vi "smart controller.vi"() -> ()   [LabVIEW 2014]
uses:
  <vilib>/Instr/_visa.llb/VISA Configure Serial Port (Instr).vi
  Environmental Chamber LabVIEW and Instruments/Drivers and Software/Keithley 2100 Series/Public/Configure/Configure 2 Wire Resistance.vi
  <vilib>/Utility/file.llb/Write To Spreadsheet File (string).vi
  Environmental Chamber LabVIEW and Instruments/Drivers and Software/keithley_6430/Keithley 6430/Public/Data/Read (Single Point).vi
  Environmental Chamber LabVIEW and Instruments/Drivers and Software/LabVIEW 8.2 Drivers/keithley_24xx/Keithley 24XX/Public/Data/Read (Single Point).vi
  <vilib>/Utility/file.llb/Read From Spreadsheet File (string).vi
  Environmental Chamber LabVIEW and Instruments/Drivers and Software/keithley_24xx/Keithley 24XX/Keithley 24XX.lvlib
  Environmental Chamber LabVIEW and Instruments/Drivers and Software/keithley_6430/Keithley 6430/Keithley 6430.lvlib
  Environmental Chamber LabVIEW and Instruments/Drivers and Software/Keithley 2100 Series/Keithley 2100 Series.lvlib
panel:
  in  "Smart start":T1={"set signal change"=100.0, " Begin smart start"=FALSE, "Reference signal"=enum."Keithley 2420", " smart start running"=FALSE} {"set signal change" min=0.0 max=100.0 step=5.0 format="%#_2f"}
  out "saving data?":bool
  out "ArduinoQCM\ncluster":T2 caption="OpenQCM" {"Freq 5" format="%#_10g"; "Freq 4" format="%#_10g"; "Freq 3" format="%#_10g"; "Freq 2" format="%#_10g"; "Freq 1" format="%#_10g"}
  in  "Data logging settings":T3={"Save during sequence only"=TRUE, "Save now"=FALSE, "sec between data points"=0.0, "Current data file path"=path "", "Save sample names"={"QCM1"="aQCM2", "QCM2"="aQCM2", "QCM3"="aQCM3", "QCM4"="aQCM4", "QCM5"="aQCM5", "QCM6"="aQCM6", "SRS"="sample_SRS", "K-2420"="Keithley2420", "K-6430"="Keithley6430", "K-2100"="Keithley2100"}, "Experiment Notes"=""} {"sec between data points" min=0.0 max=30.0 format="%#_13g"}
  in  "Sequence cluster":T4={"Save sequence"=FALSE, "Clear sequence"=FALSE, "Import sequence file"=FALSE, "Tare elapsed time"=TRUE, "Run Sequence"=FALSE, "Stop program when sequence ends"=TRUE, "User-defined\nsequence"=[], "Sequence end time"="", "Sequence\npreview"=[], "Current\nstep"=0, "Jump to next step"=FALSE} caption="Sequence settings"
  in  "Pressure parameters cluster":T5={"valve % open"=100.0, "Desired pressure"=0.0, "Vapor sccm"=0.0, "Gas sccm"=0.0, "Valve mode"=enum."% Open", "Pressure Mode"=enum."Abs. pressure", "analyte partial pressure"=23.8, "Turbo pump\nauto on"=TRUE, "Valve position (%)"=0.0, "read pressure"=0.0, "read vapor flow"=0.0, "read gas flow"=0.0, "pressure chart"={"pressure"=0.0}} caption="Pressure settings" {"read gas flow" format="%#_3g"; "read vapor flow" format="%#_3g"; "read pressure" format="%#_7f"; "Valve position (%)" format="%#_3g"; "analyte partial pressure" min=0.0 max=100.0 step=5.0; "Gas sccm" min=0 max=200 step=5; "Vapor sccm" min=0 max=200 step=5; "Desired pressure" min=0.0 max=760.0 step=5.0; "valve % open" min=0.0 max=100.0 step=5.0 format="%#_2f"}
  out "J-KEM temp chart":dbl(graph)
  out "Elapsed time (min)":dbl
  out "State date/time":string caption="Start time"
  out "K-2100 (Ohm)":cluster{"Measurement":dbl}(graph) caption="K-2100 Ohm"
  out "K-6430":cluster{"Measurement":dbl}(graph)
  out "K-2420":cluster{"Resistance":sgl}(graph)
  in  "Gate time (sec)":enum16{"0.1", "1.0 ", "10"}(ring)=enum."1.0 "
  out "MHz":dbl format="%.9f"
  out "QCM plot":T6(graph)
  in  "Stop":bool
  in  "Clear all charts":bool
  out "O2 sensor output":dbl[](array[numeric]) caption="atm\nTorr"
  in  "rapidox O2 Sensor":bool
  in  "setnag O2 Pump":bool
  in  "Baud Rate 2":i32(ring)=2 items=["2400", "4800", "9600", "19200", "38400", "57600", "115200"]
  in  "Com Port":i32(ring) items=["Com 1", "Com 2", "Com 3", "Com 4", "Com 5", "Com 6", "COM 7", "COM 8", "COM 9", "COM 10", "COM 11", "COM 12", "com 13", "COM 14"]
  in  "Com Port 2":i32(ring) items=["Com 1", "Com 2", "Com 3", "Com 4", "Com 5", "Com 6", "COM 7", "COM 8", "COM 9", "COM 10", "COM 11", "COM 12", "com 13", "COM 14"]
  out "Waveform Chart":cluster{dbl}(graph)
  out "O2 Concentration (PPM)":dbl
  out "Waveform Chart 6":cluster{dbl}(graph)
  # "Currently Unused"
  # "signal changes by less than"
  # "units"
  # "Run sequence when"
  # "100%"
  # "SRS"
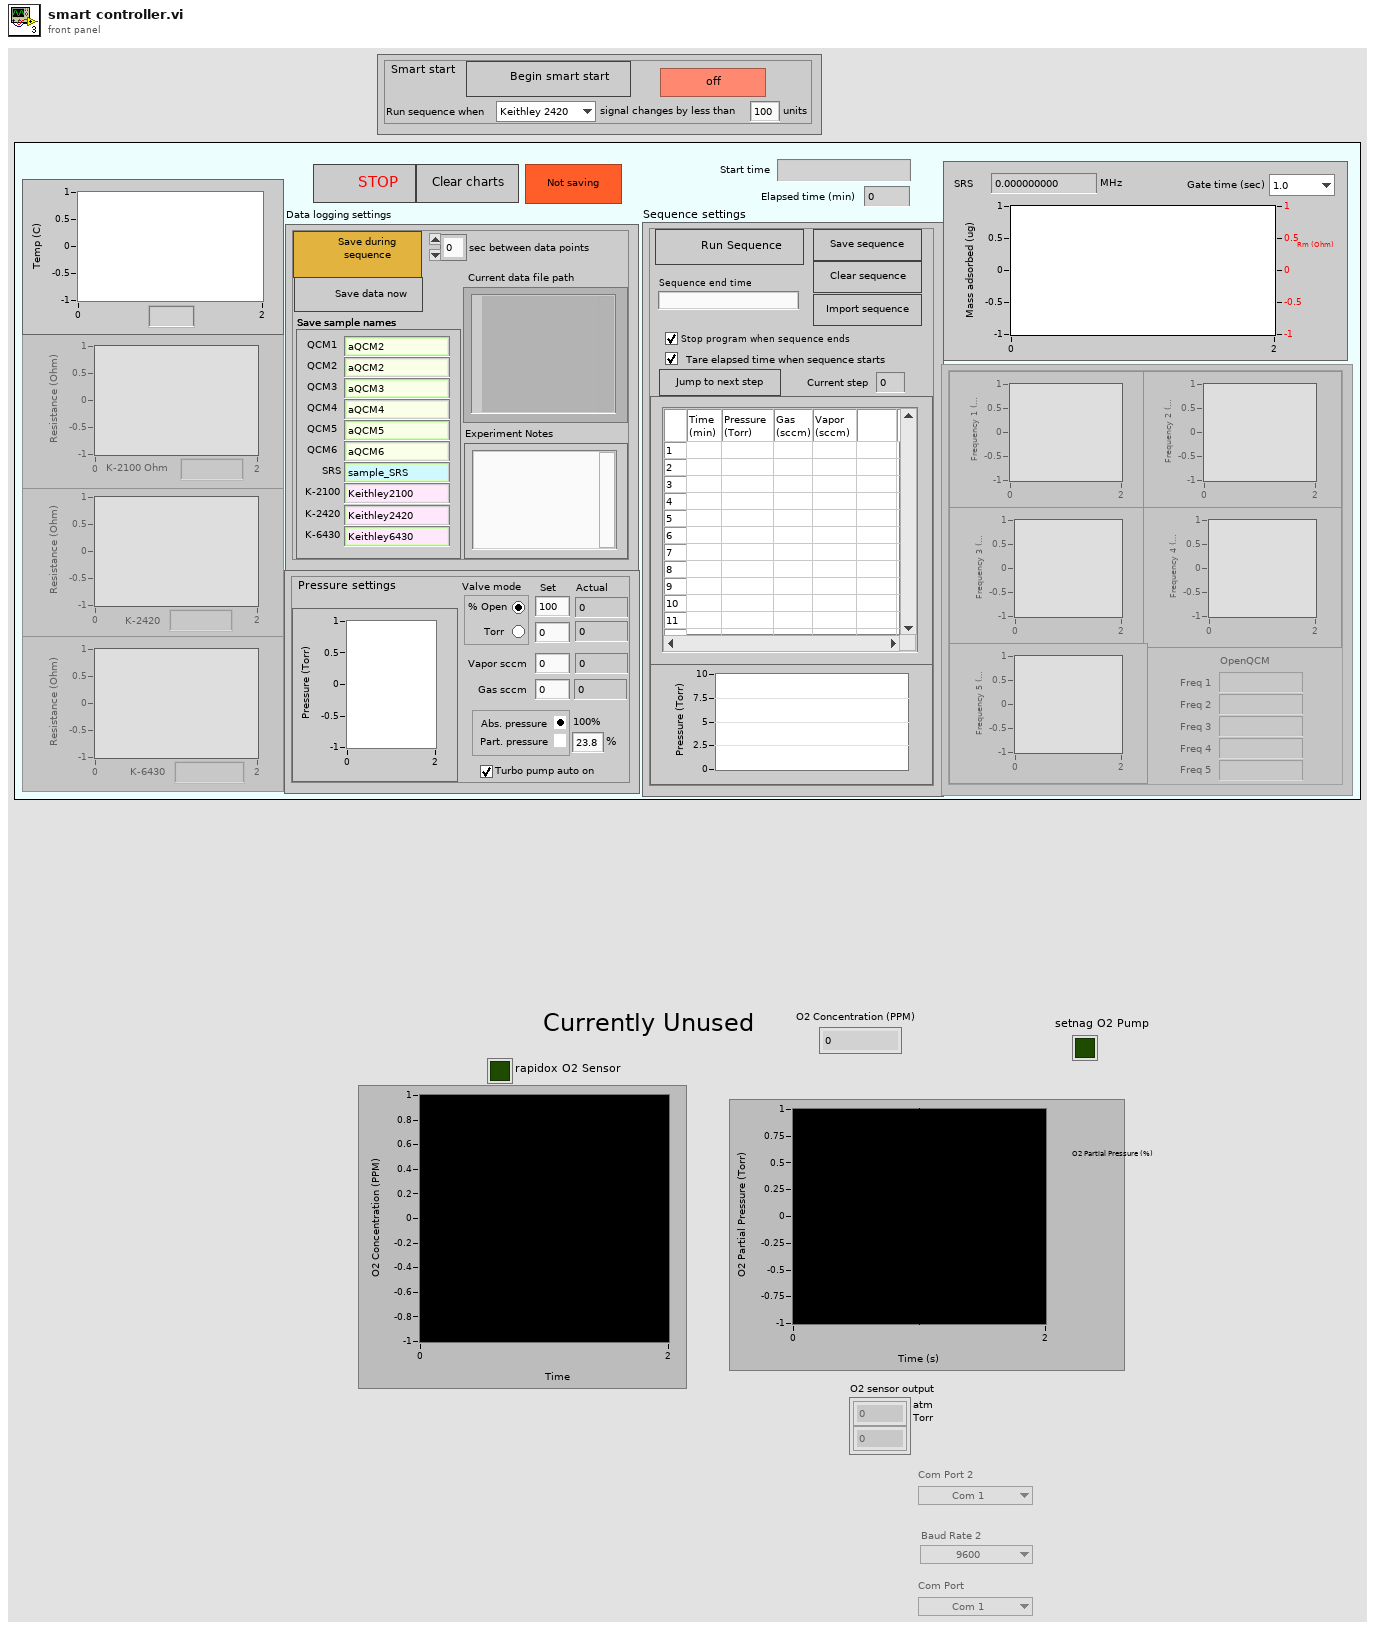
[diagram p1: front panel]
types:
  T1 = cluster{"set signal change":dbl, " Begin smart start":bool, "Reference signal":enum16{"SRS QCM", "Keithley 2420", "Keithley 6430"}, " smart start running":bool}
  T2 = cluster{"arduino qcm 1":dbl, "Freq 1":dbl, "arduino qcm 2":dbl, "Freq 2":dbl, "arduino qcm 3":dbl, "Freq 3":dbl, "arduino qcm 4":dbl, "Freq 4":dbl, "arduino qcm 5":dbl, "Freq 5":dbl}
  T3 = cluster{"Save during sequence only":bool, "Save now":bool, "sec between data points":dbl, "Current data file path":path, "Save sample names":cluster{"QCM1":string, "QCM2":string, "QCM3":string, "QCM4":string, "QCM5":string, "QCM6":string, "SRS":string, "K-2420":string, "K-6430":string, "K-2100":string}, "Experiment Notes":string}
  T4 = cluster{"Save sequence":bool, "Clear sequence":bool, "Import sequence file":bool, "Tare elapsed time":bool, "Run Sequence":bool, "Stop program when sequence ends":bool, "User-defined\nsequence":string[][], "Sequence end time":string, "Sequence\npreview":cluster{dbl[], dbl[]}[], "Current\nstep":i32, "Jump to next step":bool}
  T5 = cluster{"valve % open":dbl, "Desired pressure":dbl, "Vapor sccm":sgl, "Gas sccm":sgl, "Valve mode":enum32{"% Open", "Torr "}, "Pressure Mode":enum32{"Abs. pressure", " Part. pressure"}, "analyte partial pressure":dbl, "Turbo pump\nauto on":bool, "Valve position (%)":dbl, "read pressure":dbl, "read vapor flow":dbl, "read gas flow":dbl, "pressure chart":cluster{"pressure":dbl}}
  T6 = cluster{"Numeric Control":dbl, "Resistance out":dbl}
  T7 = cluster{"Keithley 6430":bool, "J-KEM":bool, "Keithley 2420":bool, "Keithley 2100":bool, "SRS QCM":bool, "Pressure control":bool, "Arduino":bool}
  T8 = enum8{"Enabled", "Disabled", "Disabled and Grayed Out"}
  T9 = cluster{"Arduino 1":refnum<visa-resource-name>, "Arduino 2":refnum<visa-resource-name>, "Arduino 3":refnum<visa-resource-name>, "Arduino 4":refnum<visa-resource-name>, "Arduino 5":refnum<visa-resource-name>}
  T10 = enum16{"open", "open or create", "create or replace", "create", "open (read only)"}
  T11 = enum16{"no parity", "odd parity", "even parity", "mark parity", "space parity"}
  T12 = cluster{"f":dbl, "f":dbl, "f":dbl, "f":dbl, "f":dbl}
  T13 = cluster{"String":string, "String":string, "String":string}
  T14 = cluster{"task out":refnum<k21>, "error out":errorcluster, "task out":refnum<k21>, "error out":errorcluster, "task out":refnum<k21>, "error out":errorcluster, "VISA resource name":refnum<visa-resource-name>, "error out":errorcluster}
  T15 = cluster{"task out":refnum<k21>, "error out":errorcluster, "task out":refnum<k21>, "error out":errorcluster, "task out":refnum<k21>, "error out":errorcluster, "VISA resource name out":refnum<visa-resource-name>, "error out":errorcluster}
  T16 = cluster{bool, "VISA resource name":refnum<visa-resource-name>, "error out":errorcluster}
  T17 = cluster{bool, "VISA resource name out":refnum<visa-resource-name>, "error out":errorcluster}
  T18 = cluster{"VISA resource name out":refnum<visa-resource-name>, "error out":errorcluster, "VISA resource name out":refnum<visa-resource-name>, "error out":errorcluster, "VISA resource name out":refnum<visa-resource-name>, "error out":errorcluster, "VISA resource name out":refnum<visa-resource-name>, "error out":errorcluster, "VISA resource name out":refnum<visa-resource-name>, "error out":errorcluster}
  T19 = cluster{bool, cluster{"task out":refnum<k21>, "error out":errorcluster, "task out":refnum<k21>, "error out":errorcluster, "task out":refnum<k21>, "error out":errorcluster, "VISA resource name out":refnum<visa-resource-name>, "error out":errorcluster}}
  T20 = cluster{"Boolean":bool, "VISA resource name out":refnum<visa-resource-name>, "error out":errorcluster}
  T21 = cluster{bool, "VISA out":refnum<visa-resource-name>, "error out":errorcluster}
  T22 = cluster{"Boolean":bool, "VISA out":refnum<visa-resource-name>, "error out":errorcluster}
  T23 = cluster{"Numeric Control":dbl, "Cluster":cluster{"Numeric Control":dbl}, "String":string, "error out":errorcluster}
  T24 = cluster{bool, "Com Port":i32, "Numeric Control out":dbl}
  T25 = cluster{"VISA Refnum out":refnum<visa-resource-name>, "error out":errorcluster, "VISA Refnum out":refnum<visa-resource-name>, "error out":errorcluster, "VISA Refnum out":refnum<visa-resource-name>, "error out":errorcluster, "VISA Refnum out":refnum<visa-resource-name>, "error out":errorcluster, "VISA Refnum out":refnum<visa-resource-name>, "error out":errorcluster}
  T26 = cluster{"f":string, "f":string, "f":string, "f":string, "f":string}
  T27 = cluster{"String data out":string, string, string, string}
  T28 = cluster{"valve % open":dbl, "Desired pressure":dbl, "Vapor sccm":sgl, "Gas sccm":sgl, "Valve mode":enum32{"% Open", "Torr "}, "Pressure Mode":enum32{"Abs. pressure", " Part. pressure"}, "analyte partial pressure":dbl, "Turbo pump\nauto on":bool}
  T29 = cluster{"User-defined\nsequence":string[][], "Present (s)":dbl, "current  step # in":i32, "sequence end time in":timestamp}
  T30 = cluster{"current  step # in":i32, "sequence end time in":timestamp, "Boolean":bool}
  T31 = cluster{"press/RH/gas/vapor":cluster{"pressure":string, "RH":string, "gas flow":string, "vapor flow":string}, "Cluster":cluster{"Valve position (%)":dbl, "read pressure":dbl, "read vapor flow":dbl, "read gas flow":dbl}}
  T32 = cluster{"Boolean":bool, "DAQ IDs in":cluster{"task out":refnum<k21>, "error out":errorcluster, "task out":refnum<k21>, "error out":errorcluster, "task out":refnum<k21>, "error out":errorcluster, "VISA Refnum out":refnum<visa-resource-name>, "error out":errorcluster}}
  T33 = cluster{"f":dbl, "f":dbl, "f":dbl, "f":dbl, "f":dbl}[]
  T34 = cluster{"pressure":string, "RH":string, "gas flow":string, "vapor flow":string}
  T35 = cluster{"Valve position (%)":dbl, "read pressure":dbl, "read vapor flow":dbl, "read gas flow":dbl}
  T36 = cluster{"f":dbl, "f":dbl, "f":dbl, "f":dbl, "f":dbl, "f":dbl, "f":dbl, "f":dbl, "f":dbl, "f":dbl}
  T37 = cluster{"QCM1":string, "QCM2":string, "QCM3":string, "QCM4":string, "QCM5":string, "QCM6":string, "SRS":string, "K-2420":string, "K-6430":string, "K-2100":string}
  T38 = cluster{"task out":refnum<k21>, "error out":errorcluster, "task out":refnum<k21>, "error out":errorcluster, "task out":refnum<k21>, "error out":errorcluster, "VISA Refnum out":refnum<visa-resource-name>, "error out":errorcluster}
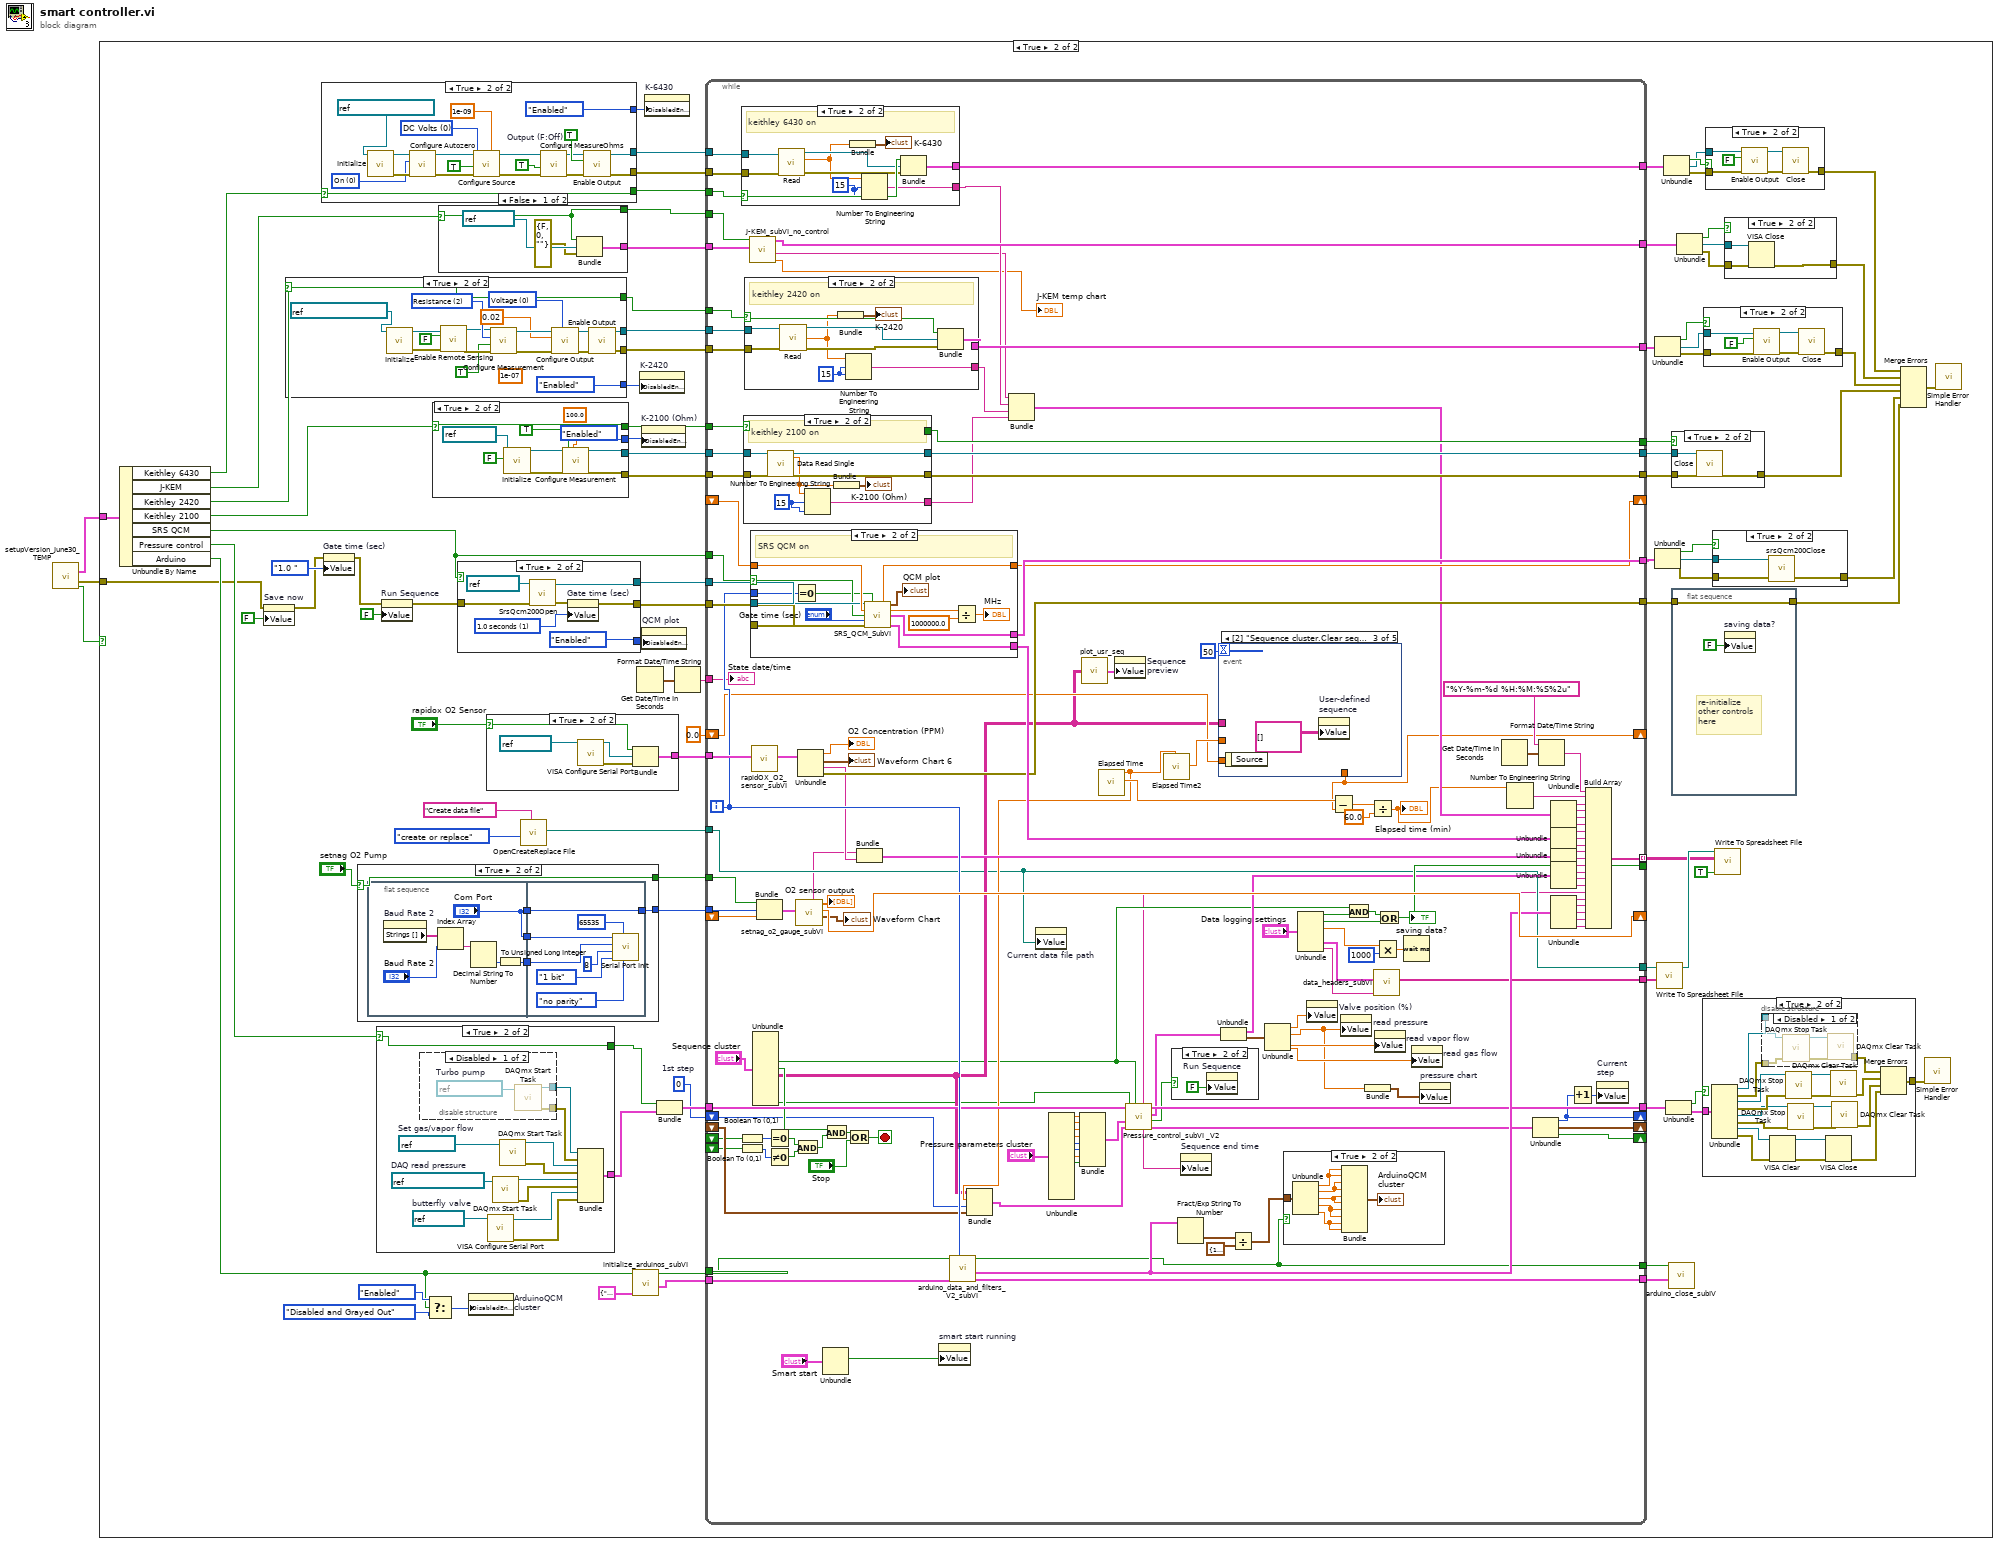
[diagram p0: block diagram]
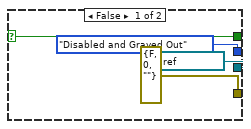
[diagram p4: hidden frame]
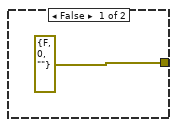
[diagram p5: hidden frame]
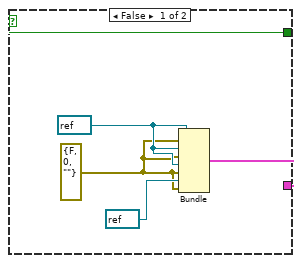
[diagram p7: hidden frame]
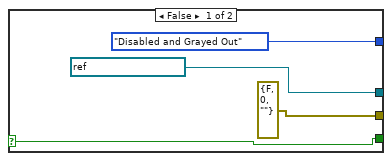
[diagram p10: hidden frame]
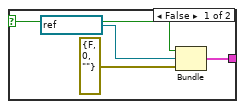
[diagram p11: hidden frame]
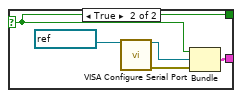
[diagram p13: hidden frame]
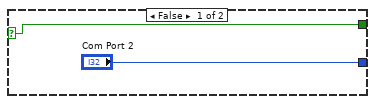
[diagram p14: hidden frame]
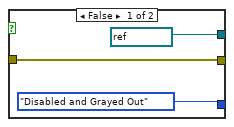
[diagram p16: hidden frame]
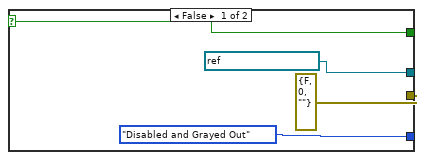
[diagram p18: hidden frame]
diagram:
  n1 = call "setupVersion_June30_TEMP.vi"() -> ("Instruments on/off"=w1:T7, "error IO"=w2:errorcluster, "OK"=w3:bool)  [unwired: 13 in]
  n2 = case shown="True" w3 {
    tunnel: w2 -> [_ w8]
    tunnel: w1 -> [_ w16]
    frame False {
    }
    frame True {
      w28 = 0  # 1st step
      n3 = Unbundle By Name(w16) -> ("Keithley 6430"=w15:bool, "J-KEM"=w14:bool, "Keithley 2420"=w13:bool, "Keithley 2100"=w12:bool, "SRS QCM"=w11:bool, "Pressure control"=w10:bool, "Arduino"=w9:bool)
      n4 = property on="Save now" class="Bool (strict)"(error in=w8, "Value"=FALSE) -> (error out=w7:errorcluster)  [unwired: 1 in, 1 out]
      n5 = case shown="True" w13 {
        selector: w13 -> [w255 w259]
        tunnel: [refnum<visa-resource-name> "GPIB1::24::INSTR" ("VISA resource name") w268] -> w92
        tunnel: [errorcluster {"status"=FALSE, "code"=0, "source"=""} ("error out") w263] -> w91
        tunnel: [T8."Disabled and Grayed Out" ("Disabled") T8."Enabled" ("Disabled")] -> w55
        tunnel: [w255 w259] -> w48
        frame False {
        }
        frame True {
          (unwired) 1e-07 ("Manual Range (1.0)")
          w270 = u16 0 items=["Voltage", "Current"] ("Source Mode  (0: Voltage)")
          w275 = u16 2 items=["Volts", "Current", "Resistance"] ("Function (0: Volts)")
          n6 = call "Initialize.vi"("VISA resource name"=refnum<visa-resource-name> "GPIB1::24::INSTR") -> ("error out"=w264:errorcluster, "VISA resource name out"=w267:refnum<visa-resource-name>)  [unwired: 9 in]
          n7 = call "Enable Remote Sensing.vi"("error in (no error)"=w264, "Enable Remote Sensing (T: Enable)"=FALSE ("4-wire?"), "VISA resource name"=w267) -> ("error out"=w265:errorcluster, "VISA resource name out"=w266:refnum<visa-resource-name>)  [unwired: 7 in]
          n8 = call "Configure Measurement.vi"("error in (no error)"=w265, "Enable Auto Range (T:Enable)"=TRUE, "Function (0: Volts)"=w275, "VISA resource name"=w266) -> ("error out"=w274:errorcluster, "VISA resource name out"=w273:refnum<visa-resource-name>)  [unwired: 6 in]
          n9 = call "Configure Output.vi"("Source Mode  (0: Voltage)"=w270, "error in (no error)"=w274, "Output Level (0)"=0.02 ("Applied Voltage (V)"), "VISA resource name"=w273) -> ("error out"=w272:errorcluster, "VISA resource name out"=w271:refnum<visa-resource-name>)  [unwired: 6 in]
          n10 = call "Enable Output.vi"("error in (no error)"=w272, "VISA resource name"=w271) -> ("error out"=w263:errorcluster, "VISA resource name out"=w268:refnum<visa-resource-name>)  [unwired: 8 in]
        }
      }
      n11 = case shown="True" w15 {
        selector: w15 -> [w169 w173]
        tunnel: [refnum<visa-resource-name> "GPIB0::29::INSTR" ("VISA resource name") w186] -> w61
        tunnel: [errorcluster {"status"=FALSE, "code"=0, "source"=""} ("error out") w187] -> w60
        tunnel: [T8."Disabled and Grayed Out" ("Disabled") T8."Enabled" ("Disabled")] -> w54
        tunnel: [w169 w173] -> w47
        frame False {
        }
        frame True {
          w175 = u16 0 items=["DC Volts", "DC Current"] ("Source Function (0: DC Volts)")
          w182 = u16 0 items=["On", "Off", "Once"] ("Autozero  (0: On)")
          w190 = TRUE  # Output (F:Off)
          n12 = call "Initialize.vi"("VISA resource name"=refnum<visa-resource-name> "GPIB0::30::INSTR") -> ("error out"=w183:errorcluster, "VISA resource name out"=w184:refnum<visa-resource-name>)  [unwired: 4 in, 5 out]
          n13 = call "Configure Autozero.vi"("error in (no error)"=w183, "Autozero  (0: On)"=w182, "VISA resource name"=w184) -> ("error out"=w178:errorcluster, "VISA resource name out"=w180:refnum<visa-resource-name>)  [unwired: 7 in]
          n14 = call "Configure Source.vi"("I-Source Level [A]"=1e-09, "error in (no error)"=w178, "Auto Range (T:Enable)"=TRUE, "Source Function (0: DC Volts)"=w175, "VISA resource name"=w180) -> ("error out"=w177:errorcluster, "VISA resource name out"=w179:refnum<visa-resource-name>)  [unwired: 5 in]
          n15 = call "Configure MeasureOhms.vi"("error in (no error)"=w177, "Auto Range (T:Enable)"=TRUE, "VISA resource name"=w179) -> ("error out"=w191:errorcluster, "VISA resource name out"=w189:refnum<visa-resource-name>)  [unwired: 3 in, 4 out]
          n16 = call "Enable Output.vi"("error in (no error)"=w191, "Enable Output (F:Off)"=w190, "VISA resource name"=w189) -> ("error out"=w187:errorcluster, "VISA resource name out"=w186:refnum<visa-resource-name>)  [unwired: 7 out]
        }
      }
      n17 = property on="Gate time (sec)" class="Enum (strict)"(error in=w7, "Value"=enum16{"0.1", "1.0 ", "10"}."1.0 " ("Gate time (sec)")) -> (error out=w17:errorcluster)  [unwired: 1 in, 1 out]
      n18 = case shown="True" "setnag O2 Pump" {
        selector: "setnag O2 Pump" -> [w214 w216]
        tunnel: ["Com Port 2" w217] -> w88
        tunnel: [w214 w216] -> w36
        frame False {
        }
        frame True {
          n19 = flat-sequence {
            tunnel: ["Com Port"] -> w220
            tunnel: [w222] -> w219
            tunnel: ["Com Port"] -> w218
            tunnel: w220 -> [w228]
            tunnel: w219 -> [w227]
            tunnel: w218 -> [w229]
            tunnel: [w229] -> w217
            frame #0 {
              n20 = property on="Baud Rate 2" class="Ring (strict)"() -> ("Strings []"=w224:string[])  [unwired: 2 in, 2 out]
              n21 = Index Array(array=w224, index="Baud Rate 2") -> (element=w225:string)
              n22 = Decimal String To Number(string=w225) -> (number=w223:i32)  [unwired: 2 in, 1 out]
              n23 = To Unsigned Long Integer(number=w223) -> (unsigned 32bit integer=w222:u32)
            }
            frame #1 {
              n24 = call <vilib>:"Serial Port Init.vi"("parity"=T11."no parity", "buffer size"=u16 65535, "stop bits"=enum16{"1 bit", "1.5 bits", "2 bits"}."1 bit", "data bits"=u16 8, "baud rate"=w227, "port number"=w228) -> ()  [unwired: 1 in, 1 out]
            }
          }
        }
      }
      n25 = case shown="True" w10 {
        selector: w10 -> [w141 w146]
        tunnel: [w142 w148] -> w30
        tunnel: [w141 w146] -> w31
        frame False {
          w144 = refnum<k21> refnum ("task out")
          w143 = errorcluster {"status"=FALSE, "code"=0, "source"=""} ("error out")
          n26 = Bundle("task out"=w144, "error out"=w143, "task out"=w144, "error out"=w143, "task out"=w144, "error out"=w143, "VISA resource name"=refnum<visa-resource-name> refnum, "error out"=w143) -> (w142:T14)  [unwired: 1 in]
        }
        frame True {
          w156 = refnum<visa-resource-name> "COM5"  # butterfly valve
          w157 = refnum<k21> "Setflow"  # Set gas/vapor flow
          w158 = refnum<k21> "AllDaqReadings"  # DAQ read pressure
          n27 = disable-structure shown="Disabled" {
            disable-tunnel: [w160 _] -> w155
            disable-tunnel: [w159 _] -> w154
            frame Disabled {
              w161 = refnum<k21> "TurboON"  # Turbo pump
              n28 = call <vilib>:"DAQmx Start Task.vi"("task/channels in"=w161) -> ("task out"=w160:refnum<k21>, "error out"=w159:errorcluster)  [unwired: 13 in]
            }
            frame Enabled {
            }
          }
          n29 = call-poly "VISA Configure Serial Port"("VISA resource name"=w156) -> ("VISA resource name out"=w149:refnum<visa-resource-name>, "error out"=w147:errorcluster)  [unwired: 13 in]
          n30 = call <vilib>:"DAQmx Start Task.vi"("task/channels in"=w158) -> ("task out"=w151:refnum<k21>, "error out"=w150:errorcluster)  [unwired: 13 in]
          n31 = call <vilib>:"DAQmx Start Task.vi"("task/channels in"=w157) -> ("task out"=w153:refnum<k21>, "error out"=w152:errorcluster)  [unwired: 13 in]
          n32 = Bundle("task out"=w155, "error out"=w154, "task out"=w153, "error out"=w152, "task out"=w151, "error out"=w150, "VISA resource name out"=w149, "error out"=w147) -> (w148:T15)  [unwired: 1 in]
        }
      }
      n33 = property on="Run Sequence" class="Bool (strict)"(error in=w17, "Value"=FALSE) -> (error out=w23:errorcluster)  [unwired: 1 in, 1 out]
      n34 = Select(t=T8."Enabled" ("Disabled"), s=w9, f=T8."Disabled and Grayed Out" ("Disabled")) -> (s? t:f=w22:T8)
      n35 = case shown="True" w12 {
        selector: w12 -> [w102 w108]
        tunnel: [refnum<visa-resource-name> "K-2100" ("VISA resource name out") w111] -> w45
        tunnel: [errorcluster {"status"=FALSE, "code"=0, "source"=""} ("error out") w110] -> w44
        tunnel: [w102 w108] -> w43
        tunnel: [T8."Disabled and Grayed Out" ("Disabled") T8."Enabled" ("Disabled")] -> w38
        frame False {
        }
        frame True {
          n36 = call "Initialize.vi"("VISA resource name"=refnum<visa-resource-name> "K-2100", "Reset? (T: Reset)"=FALSE) -> ("VISA resource name out"=w112:refnum<visa-resource-name>, "error out"=w109:errorcluster)  [unwired: 16 in]
          n37 = call-poly "Configure Measurement.vi"("VISA resource name"=w112, "error in (no error)"=w109, "Auto Range? (T: Auto)"=TRUE, "Custom Range (100 Ohm)"=100.0 ("Temp (C) 2")) -> ("VISA resource name out"=w111:refnum<visa-resource-name>, "error out"=w110:errorcluster)  [unwired: 14 in]
        }
      }
      n38 = case shown="False" w14 {
        selector: w14 -> [w205 w210]
        tunnel: [w206 w211] -> w77
        tunnel: [w205 w210] -> w71
        frame False {
          n39 = Bundle(w205, "VISA resource name"=refnum<visa-resource-name> "COM3", "error out"=errorcluster {"status"=FALSE, "code"=0, "source"=""}) -> (w206:T16)  [unwired: 1 in]
        }
        frame True {
          n40 = call-poly "VISA Configure Serial Port"("VISA resource name"=refnum<visa-resource-name> "COM3") -> ("VISA resource name out"=w212:refnum<visa-resource-name>, "error out"=w209:errorcluster)  [unwired: 13 in]
          n41 = Bundle(w210, "VISA resource name out"=w212, "error out"=w209) -> (w211:T17)  [unwired: 1 in]
        }
      }
      n42 = case shown="True" w11 {
        tunnel: [refnum<visa-resource-name> "COM6" ("VISA in") w244] -> w90
        tunnel: [w239 w241] -> w89
        tunnel: w23 -> [w239 w246]
        tunnel: [T8."Disabled and Grayed Out" ("Disabled") T8."Enabled" ("Disabled")] -> w56
        frame False {
        }
        frame True {
          w243 = u16 1 items=["0.1 seconds", "1.0 seconds", "10.0 seconds"] ("Gate time")
          n43 = call "SrsQcm200Open.vi"("error in"=w246, "VISA in"=refnum<visa-resource-name> "COM6") -> ("error out"=w242:errorcluster, "VISA out"=w244:refnum<visa-resource-name>)  [unwired: 3 in]
          n44 = property on="Gate time (sec)" class="Enum (strict)"(error in=w242, "Value"=w243) -> (error out=w241:errorcluster)  [unwired: 1 in, 1 out]
        }
      }
      n45 = property on="ArduinoQCM\ncluster" class="Clust (strict)"("DisabledEnum"=w22) -> ()  [unwired: 2 in, 2 out]
      n46 = case shown="True" "rapidox O2 Sensor" {
        selector: "rapidox O2 Sensor" -> [w192 w197]
        tunnel: [w193 w198] -> w67
        frame False {
          n47 = Bundle(w192, "VISA resource name"=refnum<visa-resource-name> "COM7", "error out"=errorcluster {"status"=FALSE, "code"=0, "source"=""}) -> (w193:T16)  [unwired: 1 in]
        }
        frame True {
          n48 = call-poly "VISA Configure Serial Port"("VISA resource name"=refnum<visa-resource-name> "COM7") -> ("VISA resource name out"=w199:refnum<visa-resource-name>, "error out"=w196:errorcluster)  [unwired: 13 in]
          n49 = Bundle(w197, "VISA resource name out"=w199, "error out"=w196) -> (w198:T17)  [unwired: 1 in]
        }
      }
      n50 = call "OpenCreateReplace File.vi"("prompt"="Create data file", "function (open:0)"=T10."create or replace") -> ("new file path"=w46:path)  [unwired: 6 in, 3 out]
      n51 = call "initialize_arduinos_subVI.vi"("arduino 1-6 addresses"=T9 {"Arduino 1"="COM21", "Arduino 2"="COM22", "Arduino 3"="COM23", "Arduino 4"="COM24", "Arduino 5"="COM26"}, "arduinos on?"=w9) -> ("arduino addresses/errors"=w32:T18, "arduinos on/off"=w52:bool)  [unwired: 8 in]
      n52 = Get Date/Time In Seconds() -> (seconds since 1Jan1904=w94:timestamp)
      n53 = property on="K-2420" class="WFChart (strict)"("DisabledEnum"=w55) -> ()  [unwired: 2 in, 2 out]
      n54 = property on="K-2100 (Ohm)" class="WFChart (strict)"("DisabledEnum"=w38) -> ()  [unwired: 2 in, 2 out]
      n55 = property on="QCM plot" class="WFChart (strict)"("DisabledEnum"=w56) -> ()  [unwired: 2 in, 2 out]
      n56 = property on="K-6430" class="WFChart (strict)"("DisabledEnum"=w54) -> ()  [unwired: 2 in, 2 out]
      n57 = Bundle(w31, w30) -> (w29:T19)  [unwired: 1 in]
      n58 = Format Date/Time String(seconds (now)=w94) -> (date/time string=w35:string)  [unwired: 2 in]
      n59 = while {
        shift-right: [w423] -> _
        shift-left: _ -> [w345]
        tunnel: [w407] -> w53 mode=indexing if=w371
        tunnel: w48 -> [w412]
        tunnel: w92 -> [w422]
        tunnel: w91 -> [w421]
        tunnel: w90 -> [w420]
        tunnel: w89 -> [w419]
        tunnel: w11 -> [w418]
        tunnel: w36 -> [w347]
        tunnel: w88 -> [w348]
        tunnel: [w417] -> w85
        tunnel: [w416] -> w81
        tunnel: w77 -> [w415]
        tunnel: [w414] -> w76
        tunnel: w71 -> [w413]
        tunnel: w67 -> [w359]
        tunnel: [w355] -> w5
        tunnel: [w287] -> w66
        tunnel: w46 -> [w287]
        shift-right: [w405] -> _
        shift-left: _ -> [w406]
        tunnel: w61 -> [w411]
        tunnel: w60 -> [w410]
        tunnel: [w409] -> w59
        tunnel: [w371] -> _
        tunnel: w52 -> [w354]
        tunnel: w32 -> [w398]
        tunnel: [w353] -> w50
        tunnel: [w397] -> w51
        tunnel: [w390] -> w49
        tunnel: w47 -> [w383]
        tunnel: w45 -> [w370]
        tunnel: w44 -> [w369]
        tunnel: w43 -> [w368]
        tunnel: [w367] -> w42
        tunnel: [w366] -> w41
        tunnel: [w365] -> w40
        shift-right: [w339] -> _
        shift-left: 0.0 ("Elapsed Time (s)") -> [w340]
        tunnel: w35 -> [w330]
        tunnel: w29 -> [w312]
        shift-right: [w282] -> _
        shift-left: w28 -> [w301]
        shift-right: [w307] -> _
        shift-left: _ -> [w305]
        shift-right: [w306] -> _
        shift-left: _ -> [w304]
        shift-left: _ -> [w303]
        tunnel: [w299] -> w27
        i -> [w349]
        stop <- w373 stop-if-true
        n60 = Boolean To (0,1)(Boolean=w304) -> (0, 1=w381:i16)
        n61 = Boolean To (0,1)(Boolean=w303) -> (0, 1=w380:i16)
        n62 = case "Keithley 6430" shown="True" w383 {
          selector: w383 -> [w457 w468]
          tunnel: w411 -> [w456 w465]
          tunnel: w410 -> [w455 w464]
          tunnel: ["" w467] -> w352
          tunnel: [w454 w466] -> w409
          frame False {
            # "keithley 6430 off"
            n63 = Bundle(w457, "VISA resource name out"=w456, "error out"=w455) -> (w454:T17)  [unwired: 1 in]
          }
          frame True {
            w459 = i16 15 ("width (-)")
            # "keithley 6430 on"
            n64 = call-poly "Read.vi"("error in (no error)"=w464, "VISA resource name"=w465) -> ("error out"=w463:errorcluster, "Measurement"=w461:dbl, "VISA resource name out"=w462:refnum<visa-resource-name>)  [unwired: 1 in, 6 out]
            n65 = Bundle("Measurement"=w461) -> (→"K-6430":cluster{"Measurement":dbl})  [unwired: 1 in]
            n66 = Number To Engineering String(2:w459, 3:w459, 4:w461) -> (0:w467:string)  [unwired: 1 in]
            n67 = Bundle(w468, "VISA resource name out"=w462, "error out"=w463) -> (w466:T17)  [unwired: 1 in]
          }
        }
        n68 = case shown="True" w368 {
          selector: w368 -> [w433 w438]
          tunnel: [w434 w445] -> w366
          tunnel: [w435 w444] -> w365
          tunnel: w370 -> [w434 w443]
          tunnel: w369 -> [w435 w442]
          tunnel: ["" w440] -> w350
          tunnel: [w433 w438] -> w367
          frame False {
            # "keithley 2100 off"
          }
          frame True {
            w437 = i16 15 ("width (-)")
            # "keithley 2100 on"
            n69 = call "Data Read Single.vi"("VISA resource name"=w443, "error in (no error)"=w442) -> ("VISA resource name out"=w445:refnum<visa-resource-name>, "Measurement"=w441:dbl, "error out"=w444:errorcluster)  [unwired: 15 in]
            n70 = Number To Engineering String ("elapsed time (min)")(2:w437, 3:w437, 4:w441) -> (0:w440:string)  [unwired: 1 in]
            n71 = Bundle("Measurement"=w441) -> (→"K-2100 (Ohm)":cluster{"Measurement":dbl})  [unwired: 1 in]
          }
        }
        n72 = case "Keithley 2420" shown="True" w412 {
          selector: w412 -> [w472 w481]
          tunnel: w422 -> [w471 w476]
          tunnel: w421 -> [w470 w475]
          tunnel: [w469 w479] -> w417
          tunnel: ["" w478] -> w351
          frame False {
            # "keithley 2420 off"
            n73 = Bundle(w472, "VISA resource name out"=w471, "error out"=w470) -> (w469:T17)  [unwired: 1 in]
          }
          frame True {
            w474 = i16 15 ("width (-)")
            # "keithley 2420 on"
            n74 = call-poly "Read.vi"("VISA resource name"=w476, "error in (no error)"=w475) -> ("VISA resource name out"=w482:refnum<visa-resource-name>, "Resistance"=w477:sgl, "error out"=w480:errorcluster)  [unwired: 7 in, 4 out]
            n75 = Bundle("Resistance"=w477) -> (→"K-2420":cluster{"Resistance":sgl})  [unwired: 1 in]
            n76 = Number To Engineering String(2:w474, 3:w474, 4:w477) -> (0:w478:string)  [unwired: 1 in]
            n77 = Bundle(w481, "VISA resource name out"=w482, "error out"=w480) -> (w479:T17)  [unwired: 1 in]
          }
        }
        n78 = call "J-KEM_subVI_no_control.vi"("Address in"=w415, "J-KEM on?"=w413) -> ("Temp (C)"=→"J-KEM temp chart":dbl, "String data out"=w338:string, "Address out"=w414:T20)  [unwired: 6 in, 1 out]
        n79 = case "SRS QCM" shown="True" w418 {
          selector: w418 -> [w486 w497]
          tunnel: w420 -> [w489 w499]
          tunnel: w419 -> [w488 w500]
          tunnel: [w487 w503] -> w416
          tunnel: w406 -> [w484 w502]
          tunnel: [w484 w501] -> w405
          tunnel: [T13 {"String"="", "String"="", "String"=""} ("M,F,MR output cluster") w496] -> w395
          tunnel: w349 -> [_ w490]
          frame False {
            # "SRS QCM off"
            n80 = Bundle(w486, "VISA out"=w489, "error out"=w488) -> (w487:T21)  [unwired: 1 in]
          }
          frame True {
            # "SRS QCM on"
            n81 = Equal To 0?(x=w490) -> (x = 0?=w491:bool)
            n82 = call "SRS_QCM_SubVI.vi"("VISA Refnum in"=w499, "first iteration?"=w491, "Frequency out 3"=w502, "Boolean 2"=w497, "Gate time"="Gate time (sec)", "error in (no error)"=w500) -> ("Frequency out 2"=w501:dbl, "Cluster"=→"QCM plot":T6, "Frequency out"=w492:dbl, "Cluster 2"=w503:T22, "M,F,MR output cluster"=w496:T13)  [unwired: 2 in, 3 out]
            n83 = Divide(x=w492, y=1000000.0) -> (x/y=→"MHz":dbl)
          }
        }
        n84 = call "rapidOX_O2_sensor_subVI.vi"("rapid ox info in"=w359) -> ("rapidox info out"=w358:T23)  [unwired: 10 in]
        n85 = Unbundle("Sequence cluster") -> ("Run Sequence"=w293:bool, "Stop program when sequence ends"=w302:bool, "User-defined\nsequence"=w297:string[][], "Jump to next step"=w283:bool)  [unwired: 7 out]
        n86 = Bundle(w347, "Com Port"=w348, "Numeric Control out"=w345) -> (w346:T24)  [unwired: 1 in]
        n87 = Equal To 0?(x=w381) -> (x = 0?=w378:bool)
        n88 = Not Equal To 0?(x=w380) -> (x != 0?=w379:bool)
        n89 = And(x=w378, y=w379) -> (x .and. y?=w372:bool)
        n90 = call "setnag_o2_gauge_subVI.vi"("setnag info in"=w346) -> ("Cluster"=→"Waveform Chart":cluster{"Numeric Control":dbl}, "Numeric Control out"=w423:dbl, "Array"=→"O2 sensor output":dbl[], "String"=w284:string)  [unwired: 7 in]
        n91 = Unbundle(w358) -> ("Numeric Control"=→"O2 Concentration (PPM)":dbl, "Cluster"=→"Waveform Chart 6":cluster{"Numeric Control":dbl}, "String"=w329:string, "error out"=w355:errorcluster)
        n92 = Unbundle("Smart start") -> ("Begin smart start"=w277:bool)  [unwired: 3 out]
        n93 = And(x=w302, y=w372) -> (x .and. y?=w343:bool)
        n94 = Or(x=w343, y="Stop") -> (x .or. y?=w373:bool)
        n95 = Bundle("String"=w284, "String"=w329) -> (w328:cluster{"String":string, "String":string})  [unwired: 1 in]
        n96 = property on="smart start running" class="Bool (strict)"("Value"=w277) -> ()  [unwired: 2 in, 2 out]
        n97 = call "arduino_data_and_filters_V2_subVI.vi"("loop iteration number"=w349, "arduino 1-6 address and errors"=w398, "arduinos on?"=w354) -> ("arduino 1-6 addresses and errors out"=w397:T25, "arduino 1-6 data out"=w396:T26, "arduinos on? output"=w353:bool)  [unwired: 6 in]
        n98 = Bundle("String data out"=w338, w352, w351, w350) -> (w344:T27)  [unwired: 1 in]
        n99 = property on="Current data file path" class="Path"("Value"=w287) -> ()  [unwired: 2 in, 2 out]
        n100 = Unbundle("Pressure parameters cluster") -> ("valve % open"=w317:dbl, "Desired pressure"=w319:dbl, "Vapor sccm"=w320:sgl, "Gas sccm"=w321:sgl, "Valve mode"=w322:enum32{"% Open", "Torr "}, "Pressure Mode"=w323:enum32{"Abs. pressure", " Part. pressure"}, "analyte partial pressure"=w324:dbl, "Turbo pump\nauto on"=w325:bool)  [unwired: 5 out]
        n101 = Bundle("valve % open"=w317, "Desired pressure"=w319, "Vapor sccm"=w320, "Gas sccm"=w321, "Valve mode"=w322, "Pressure Mode"=w323, "analyte partial pressure"=w324, "Turbo pump\nauto on"=w325) -> (w316:T28)  [unwired: 1 in]
        n102 = call "plot_usr_seq.vi"("User-defined sequence"=w297) -> ("Sequence Preview"=w289:cluster{dbl[], dbl[]}[])
        n103 = call "Elapsed Time"() -> ("Present (s)"=w309:dbl, "Elapsed Time (s)"=w361:dbl)  [unwired: 12 in, 6 out]
        n104 = Bundle("User-defined\nsequence"=w297, "Present (s)"=w309, "current  step # in"=w301, "sequence end time in"=w305) -> (w310:T29)  [unwired: 1 in]
        n105 = property on="Sequence\npreview" class="XYGraph (strict)"("Value"=w289) -> ()  [unwired: 2 in, 2 out]
        n106 = call "Pressure_control_subVI _V2.vi"("Run Sequence"=w293, "user sequence, present (s) in, current step in, seq time in"=w310, "pressure parameters in"=w316, "Jump to next step"=w283, "pressure control on? / DAQ IDs/errors in"=w312) -> ("current step # out, shift register time out, seq button on?"=w308:T30, "sequence over? USE THIS TO REINITIALIZE RUN SEQUENCE BUTTON SO PROGRAM ENDS"=w298:bool, "save press/RH/gasflow/vaporflow - read valve position/pressure/vaporflow/gasflow"=w296:T31, "pressure control on out, DAQ IDs/errors out"=w299:T32, "sequence end date/time string"=w300:string, "pressure_setpoint"=w279:string)  [unwired: 1 in]
        n107 = call "Elapsed Time2"("Set Start Time (s)"=w309) -> ("Elapsed Time (s)"=w341:dbl)  [unwired: 11 in, 7 out]
        n108 = case shown="True" w298 {
          frame False {
          }
          frame True {
            n109 = property on="Run Sequence" class="Bool (strict)"("Value"=FALSE ("Run Sequence")) -> ()  [unwired: 2 in, 2 out]
          }
        }
        n110 = Fract/Exp String To Number(string=w396) -> (number=w389:T12)  [unwired: 3 in, 1 out]
        n111 = property on="Sequence end time" class="Str"("Value"=w300) -> ()  [unwired: 2 in, 2 out]
        n112 = event shown="[2] \"Sequence cluster.Clear sequence\": Value Change" {
          selector: _ -> [_ _ _ _ _]
          dyn-events: _ -> [_ _ _ _ _]
          timeout: 50 -> [_ _ _ _ _]
          tunnel: w297 -> [_ _ _ w452 _]
          tunnel: w341 -> [_ _ _ _ _]
          tunnel: w340 -> [w446 _ _ _ _]
          tunnel: [w446 _ _ _ _] -> w339
          event Timeout {
            n113 = event-data() -> ()  [unwired: 1 in, 1 out]
          }
          event "Clear all charts": Value Change {
            (unwired) T33 [] ("History Data")
            w449 = cluster{dbl}[] [] ("History Data")
            w450 = cluster{"Resistance":sgl}[] [] ("History Data")
            w448 = dbl[] [] ("History Data")
            n114 = event-data() -> ()  [unwired: 1 in, 1 out]
            n115 = property on="K-6430" class="WFChart (strict)"("History Data"=w450) -> ()  [unwired: 2 in, 2 out]
            n116 = property on="arduino qcm 3" class="WFChart (strict)"("History Data"=w448) -> ()  [unwired: 2 in, 2 out]
            n117 = property on="arduino qcm 1" class="WFChart (strict)"("History Data"=w448) -> ()  [unwired: 2 in, 2 out]
            n118 = property on="Waveform Chart" class="WFChart (strict)"("History Data"=w449) -> ()  [unwired: 2 in, 2 out]
            n119 = property on="QCM plot" class="WFChart (strict)"("History Data"=cluster{dbl, "Resistance out":dbl}[] []) -> ()  [unwired: 2 in, 2 out]
            n120 = property on="K-2100 (Ohm)" class="WFChart (strict)"("History Data"=w450) -> ()  [unwired: 2 in, 2 out]
            n121 = property on="arduino qcm 4" class="WFChart (strict)"("History Data"=w448) -> ()  [unwired: 2 in, 2 out]
            n122 = property on="K-2420" class="WFChart (strict)"("History Data"=w450) -> ()  [unwired: 2 in, 2 out]
            n123 = property on="pressure chart" class="WFChart (strict)"("History Data"=w449) -> ()  [unwired: 2 in, 2 out]
            n124 = property on="arduino qcm 2" class="WFChart (strict)"("History Data"=w448) -> ()  [unwired: 2 in, 2 out]
            n125 = property on="arduino qcm 5" class="WFChart (strict)"("History Data"=w448) -> ()  [unwired: 2 in, 2 out]
          }
          event "Sequence cluster.Clear sequence": Value Change {
            n126 = event-data() -> ()  [unwired: 1 in, 1 out]
            n127 = property on="User-defined\nsequence" class="Tbl (strict)"("Value"=string[][] []) -> ()  [unwired: 2 in, 2 out]
          }
          event "Sequence cluster.Save sequence": Value Change {
            n128 = event-data() -> ()  [unwired: 1 in, 1 out]
            n129 = call-poly <vilib>:"Write To Spreadsheet File.vi"("2D data"=w452) -> ()  [unwired: 7 in, 1 out]
          }
          event "Sequence cluster.Import sequence file": Value Change {
            n130 = event-data() -> ()  [unwired: 1 in, 1 out]
            n131 = call-poly <vilib>:"Read From Spreadsheet File.vi"() -> ("all rows"=w453:string[][])  [unwired: 7 in, 4 out]
            n132 = property on="User-defined\nsequence" class="Tbl (strict)"("Value"=w453) -> ()  [unwired: 2 in, 2 out]
          }
        }
        n133 = Unbundle(w296) -> ("press/RH/gas/vapor"=w295:T34, "Cluster"=w294:T35)
        n134 = Divide(x=w389, y=T12 {"f"=1000000.0, "f"=1000000.0, "f"=1000000.0, "f"=1000000.0, "f"=1000000.0}) -> (x/y=w364:T12)
        n135 = Unbundle(w294) -> ("Valve position (%)"=w292:dbl, "read pressure"=w286:dbl, "read vapor flow"=w291:dbl, "read gas flow"=w290:dbl)
        n136 = case shown="True" w353 {
          tunnel: w364 -> [_ w432]
          frame False {
          }
          frame True {
            n137 = Unbundle(w432) -> ("f"=w431:dbl, "f"=w430:dbl, "f"=w429:dbl, "f"=w428:dbl, "f"=w427:dbl)
            n138 = Bundle("f"=w431, "f"=w431, "f"=w430, "f"=w430, "f"=w429, "f"=w429, "f"=w428, "f"=w428, "f"=w427, "f"=w427) -> (→"ArduinoQCM\ncluster":T36)  [unwired: 1 in]
          }
        }
        n139 = Unbundle("Data logging settings") -> ("Save during sequence only"=w375:bool, "Save now"=w377:bool, "sec between data points"=w363:dbl, "Save sample names"=w314:T37, "Experiment Notes"=w313:string)  [unwired: 1 out]
        n140 = property on="Valve position (%)" class="DigNum (strict)"("Value"=w292) -> ()  [unwired: 2 in, 2 out]
        n141 = Subtract(x=w361, y=w339) -> (x-y=w360:dbl)
        n142 = property on="read pressure" class="DigNum (strict)"("Value"=w286) -> ()  [unwired: 2 in, 2 out]
        n143 = And(x=w293, y=w375) -> (x .and. y?=w374:bool)
        n144 = Bundle("read pressure"=w286) -> (w285:cluster{"read pressure":dbl})  [unwired: 1 in]
        n145 = Divide(x=w360, y=60.0) -> (x/y=w331:dbl)
        "Elapsed time (min)" <- w331
        n146 = call "data_headers_subVI.vi"("Experiment Notes"=w313, "Sample names"=w314) -> ("data headers"=w390:string[])  [unwired: 9 in]
        n147 = property on="read vapor flow" class="DigNum (strict)"("Value"=w291) -> ()  [unwired: 2 in, 2 out]
        n148 = Multiply(x=w363, y=u32 1000 ("x")) -> (x*y=w402:dbl)
        n149 = Or(x=w374, y=w377) -> (x .or. y?=w371:bool)
        "saving data?" <- w371
        n150 = Wait (ms)(milliseconds to wait=w402) -> ()  [unwired: 1 out]
        n151 = property on="read gas flow" class="DigNum (strict)"("Value"=w290) -> ()  [unwired: 2 in, 2 out]
        n152 = property on="pressure chart" class="WFChart (strict)"("Value"=w285) -> ()  [unwired: 2 in, 2 out]
        n153 = Get Date/Time In Seconds() -> (seconds since 1Jan1904=w424:timestamp)
        n154 = Number To Engineering String ("elapsed time (min)")(4:w331) -> (0:w336:string)  [unwired: 3 in]
        n155 = Unbundle(w308) -> ("current  step # in"=w282:i32, "sequence end time in"=w307:timestamp, "Boolean"=w306:bool)
        n156 = Format Date/Time String(time format string (%c)="%Y-%m-%d %H:%M:%S%2u", seconds (now)=w424) -> (date/time string=w399:string)  [unwired: 1 in]
        n157 = Unbundle(w344) -> ("String data out"=w335:string, w334:string, w333:string, w332:string)
        n158 = Unbundle(w395) -> ("String"=w337:string, "String"=w401:string, "String"=w400:string)
        n159 = Unbundle(w328) -> ("String"=w327:string, "String"=w326:string)
        n160 = Unbundle(w295) -> ("pressure"=w387:string, "RH"=w386:string, "gas flow"=w385:string, "vapor flow"=w384:string)
        n161 = Unbundle ("arduino 1-6")(w396) -> ("f"=w280:string, "f"=w394:string, "f"=w393:string, "f"=w392:string, "f"=w391:string)
        n162 = Increment(x=w282) -> (x+1=w281:i32)
        n163 = Build Array(w399, w336, w335, w334, w333, w332, w337, w401, w400, w327, w326, w387, w386, w385, w384, w279, w280, w394, w393, w392, w391) -> (w407:string[])
        n164 = property on="Current\nstep" class="DigNum (strict)"("Value"=w281) -> ()  [unwired: 2 in, 2 out]
        "State date/time" <- w330
      }
      n165 = Unbundle(w85) -> (w84:bool, "VISA resource name out"=w83:refnum<visa-resource-name>, "error out"=w82:errorcluster)
      n166 = Unbundle(w81) -> ("Boolean"=w80:bool, "VISA out"=w79:refnum<visa-resource-name>, "error out"=w78:errorcluster)
      n167 = call-poly <vilib>:"Write To Spreadsheet File.vi"("1D data"=w49, "file path (dialog if empty)"=w66) -> ("new file path (Not A Path if cancelled)"=w70:path)  [unwired: 6 in]
      n168 = Unbundle(w59) -> (w64:bool, "VISA resource name out"=w63:refnum<visa-resource-name>, "error out"=w62:errorcluster)
      n169 = Unbundle(w27) -> ("Boolean"=w26:bool, "DAQ IDs in"=w25:T38)
      n170 = call "arduino_close_subIV.vi"("arduino 1-6 addresses and errors out"=w51, "arduinos on?"=w50) -> ()  [unwired: 10 in]
      n171 = case shown="True" w42 {
        tunnel: w41 -> [_ w100]
        tunnel: w40 -> [w97 w99]
        tunnel: [w97 w98] -> w39
        frame False {
        }
        frame True {
          n172 = call "Close.vi"("VISA resource name"=w100, "error in (no error)"=w99) -> ("error out"=w98:errorcluster)  [unwired: 17 in]
        }
      }
      n173 = flat-sequence {
        tunnel: w5 -> [w96]
        tunnel: [w96] -> w4
        frame #0 {
          # "re-initialize \nother controls\nhere"
          n174 = property on="saving data?" class="Bool (strict)"("Value"=FALSE ("saving data?")) -> ()  [unwired: 2 in, 2 out]
        }
      }
      n175 = Unbundle(w76) -> ("Boolean"=w75:bool, "VISA resource name out"=w74:refnum<visa-resource-name>, "error out"=w73:errorcluster)
      n176 = case shown="True" w26 {
        tunnel: w25 -> [_ w129]
        tunnel: [errorcluster {"status"=FALSE, "code"=0, "source"=""} ("error out") w116] -> w34
        frame False {
        }
        frame True {
          n177 = Unbundle(w129) -> ("task out"=w128:refnum<k21>, "error out"=w127:errorcluster, "task out"=w126:refnum<k21>, "error out"=w125:errorcluster, "task out"=w124:refnum<k21>, "error out"=w123:errorcluster, "VISA Refnum out"=w122:refnum<visa-resource-name>, "error out"=w121:errorcluster)
          n178 = disable-structure shown="Disabled" {
            disable-tunnel: [w138 _] -> w120
            disable-tunnel: w128 -> [w137 _]
            disable-tunnel: w127 -> [w136 _]
            frame Disabled {
              n179 = call <vilib>:"DAQmx Stop Task.vi"("task/channels in"=w137, "error in"=w136) -> ("task out"=w139:refnum<k21>, "error out"=w140:errorcluster)  [unwired: 12 in]
              n180 = call <vilib>:"DAQmx Clear Task.vi"("task in"=w139, "error in"=w140) -> ("error out"=w138:errorcluster)  [unwired: 13 in]
            }
            frame Enabled {
            }
          }
          n181 = VISA Clear(VISA resource name=w122, error in (no error)=w121) -> (VISA resource name out=w131:refnum<visa-resource-name>, error out=w130:errorcluster)
          n182 = call <vilib>:"DAQmx Stop Task.vi"("task/channels in"=w126, "error in"=w125) -> ("task out"=w133:refnum<k21>, "error out"=w132:errorcluster)  [unwired: 12 in]
          n183 = call <vilib>:"DAQmx Stop Task.vi"("task/channels in"=w124, "error in"=w123) -> ("task out"=w134:refnum<k21>, "error out"=w135:errorcluster)  [unwired: 12 in]
          n184 = VISA Close(VISA resource name=w131, error in (no error)=w130) -> (error out=w117:errorcluster)
          n185 = call <vilib>:"DAQmx Clear Task.vi"("task in"=w133, "error in"=w132) -> ("error out"=w119:errorcluster)  [unwired: 13 in]
          n186 = call <vilib>:"DAQmx Clear Task.vi"("task in"=w134, "error in"=w135) -> ("error out"=w118:errorcluster)  [unwired: 13 in]
          n187 = Merge Errors(w120, w119, w118, w117) -> (w116:errorcluster)
        }
      }
      n188 = case shown="True" w84 {
        tunnel: w83 -> [_ w251]
        tunnel: w82 -> [w248 w250]
        tunnel: [w248 w249] -> w86
        frame False {
        }
        frame True {
          n189 = call "Enable Output.vi"("error in (no error)"=w250, "Enable Output (T: Enable)"=FALSE, "VISA resource name"=w251) -> ("error out"=w252:errorcluster, "VISA resource name out"=w254:refnum<visa-resource-name>)  [unwired: 7 in]
          n190 = call "Close.vi"("error in (no error)"=w252, "VISA resource name"=w254) -> ("error out"=w249:errorcluster)  [unwired: 9 in]
        }
      }
      n191 = case shown="True" w64 {
        tunnel: w63 -> [_ w164]
        tunnel: w62 -> [w162 w163]
        tunnel: [w162 w165] -> w58
        frame False {
        }
        frame True {
          n192 = call "Enable Output.vi"("error in (no error)"=w163, "Enable Output (F:Off)"=FALSE ("Output (F:Off)"), "VISA resource name"=w164) -> ("error out"=w166:errorcluster, "VISA resource name out"=w167:refnum<visa-resource-name>)  [unwired: 7 out]
          n193 = call "Close.vi"("error in (no error)"=w166, "VISA resource name"=w167) -> ("error out"=w165:errorcluster)  [unwired: 9 out]
        }
      }
      n194 = case shown="True" w80 {
        tunnel: w78 -> [w234 w237]
        tunnel: [w234 w236] -> w87
        tunnel: w79 -> [_ w235]
        frame False {
        }
        frame True {
          n195 = call "srsQcm200Close.vi"("error in"=w237, "Visa in"=w235) -> ("error out"=w236:errorcluster)  [unwired: 3 in]
        }
      }
      n196 = call-poly <vilib>:"Write To Spreadsheet File.vi"("append to file? (new file:F)"=TRUE, "2D data"=w53, "file path (dialog if empty)"=w70) -> ()  [unwired: 5 in, 1 out]
      n197 = case shown="True" w75 {
        tunnel: w74 -> [_ w204]
        tunnel: w73 -> [w201 w203]
        tunnel: [w201 w202] -> w72
        frame False {
        }
        frame True {
          n198 = VISA Close(VISA resource name=w204, error in (no error)=w203) -> (error out=w202:errorcluster)
        }
      }
      n199 = Merge Errors(w58, w72, w86, w39, w87, w4) -> (w93:errorcluster)
      n200 = call <vilib>:"Simple Error Handler.vi"("error in (no error)"=w34) -> ()  [unwired: 4 in, 5 out]
      n201 = call <vilib>:"Simple Error Handler.vi"("error in (no error)"=w93) -> ()  [unwired: 4 in, 5 out]
    }
  }
